vi "MAIN_HGB2.vi"() -> ()   [LabVIEW 2016]
uses:
  Producer_Case_Structure.ctl
  <vilib>/Utility/error.llb/DialogType.ctl
  <vilib>/express/express analysis/Spectral/Block/exnSpectralBlock spectral measurements RMS poly.vi
  <vilib>/express/express analysis/Spectral/Block/exnSpectralBlock spectral measurements RMS array WFM.vi
  <vilib>/express/express analysis/Spectral/XNode/ExpressSpectralMeasurementsBlockNode.xnode
panel:
  in  "Speed Setpoint":dbl
  in  "Operator Notes":string
  in  "Dummy Variable":dbl
  in  "Record Data":bool
  in  "Sample Rate [S/s]":dbl=10.0
  in  "file path":path=path "S:/002 - Projects/200804 AECSSB/6-Testing/TDMS Data/raw/080421-1"
  in  "Stop":bool=TRUE
  in  "Tab Control":T1(tab)=enum."Pressure & Temperature"
  out "System Temperatures":waveform(dbl)[](graph)=[{"t0"=timestamp(3710938237.209422 s since 1904-01-01), "dt"=0.1, "Y"=[25.06420596580779], "attributes"=variant("NI_ChannelName"=variant(string "T_dis"), "NI_UnitDescription"=variant(string "Deg C"))}, {"t0"=timestamp(3710938237.209422 s since 1904-01-01), "dt"=0.1, "Y"=[24.5131871952291], "attributes"=variant("NI_ChannelName"=variant(string "T_liq_mix"), "NI_UnitDescription"=variant(string "Deg C"))}, {"t0"=timestamp(3710938237.209422 s since 1904-01-01), "dt"=0.1, "Y"=[24.404692160048143], "attributes"=variant("NI_ChannelName"=variant(string "T_gas_mix"), "NI_UnitDescription"=variant(string "Deg C"))}, {"t0"=timestamp(3710938237.209422 s since 1904-01-01), "dt"=0.1, "Y"=[24.9517211018332], "attributes"=variant("NI_ChannelName"=variant(string "T_wf_cond_out"), "NI_UnitDescription"=variant(string "Deg C"))}, {"t0"=timestamp(3710938237.209422 s since 1904-01-01), "dt"=0.1, "Y"=[24.75846841874906], "attributes"=variant("NI_ChannelName"=variant(string "T_cf_in"), "NI_UnitDescription"=variant(string "Deg C"))}]
  out "Power Constituents":waveform(dbl)[](graph)=[{"t0"=timestamp(3710938237.209422 s since 1904-01-01), "dt"=0.1, "Y"=[-0.0627204059992863], "attributes"=variant("NI_ChannelName"=variant(string "Voltage"))}, {"t0"=timestamp(3710938237.209422 s since 1904-01-01), "dt"=0.1, "Y"=[-0.029340257114334634], "attributes"=variant("NI_ChannelName"=variant(string "Frequency"))}, {"t0"=timestamp(3710938237.0104485 s since 1904-01-01), "dt"=0.1, "Y"=[], "attributes"=variant("NI_ChannelName"=variant(string "Torque"))}]
  out "System Pressures":waveform(dbl)[](graph)=[{"t0"=timestamp(3710938237.209422 s since 1904-01-01), "dt"=0.1, "Y"=[653.0149804276925], "attributes"=variant("NI_ChannelName"=variant(string "P_comp_suc"))}, {"t0"=timestamp(3710938237.209422 s since 1904-01-01), "dt"=0.1, "Y"=[652.9848572024544], "attributes"=variant("NI_ChannelName"=variant(string "P_comp_dis"))}, {"t0"=timestamp(3710938237.209422 s since 1904-01-01), "dt"=0.1, "Y"=[653.0856354357659], "attributes"=variant("NI_ChannelName"=variant(string "P_comp_int"))}]
  out "Mass Flow":waveform(dbl)(graph)={"t0"=timestamp(3710938237.209422 s since 1904-01-01), "dt"=0.1, "Y"=[-2.0362630357040334e-05], "attributes"=variant("NI_ChannelName"=variant(string "m_dot_wf"))}
  out "Raw Acceleration":waveform(dbl)[](graph)
  out "Accel. Spectrum":cluster{"f0":dbl, "df":dbl, "magnitude":dbl[]}[](graph)
  in  "?":path=path "C:/Users/ASITest/Desktop/REFPROP"
  in  "Working Fluid":string="R134A.FLD"
  out "Sound":waveform(dbl)(graph)
  in  "Range":enum16{"40-70 dB", "auto", "60-90 dB"}(ring)
  in  "Ambient Noise [dB]":dbl=74.0
  # "Stop VI"
  # "Air Squared Hot Gas Bypass Test Stand"
  # "Point to where REFPROP is..."
  # "Registar Index of Calc Characteristics"
  # "INPUT NEEDED"
  # "0 = No\n1 = Yes"
  # "0 = No\n1 = Yes"
  # "UNITS:\nkg/s\nC\nRPM\nkPa\nV\nA"
  # "... where is the sensor in the initialization indexing?"
  # "Must have sound meter set up to manual range:\n1. click 'RNG' button on the meter \n2. the value displayed under 'SPL' on the display is the min of the range\n3. ensure the meter is on 'FAST' mode by clicking 'F/S', 'FAST' will be read on display\n4. use the A/C to select 'A' mode displayed on meter\n5. BEFORE INITIALIZING - set ambient noise level to whatever the sensor measures before running\n* the extech 407730 display frequency is not as high as the display freq here, so peak values\nmay not be seen on the sound meter display."
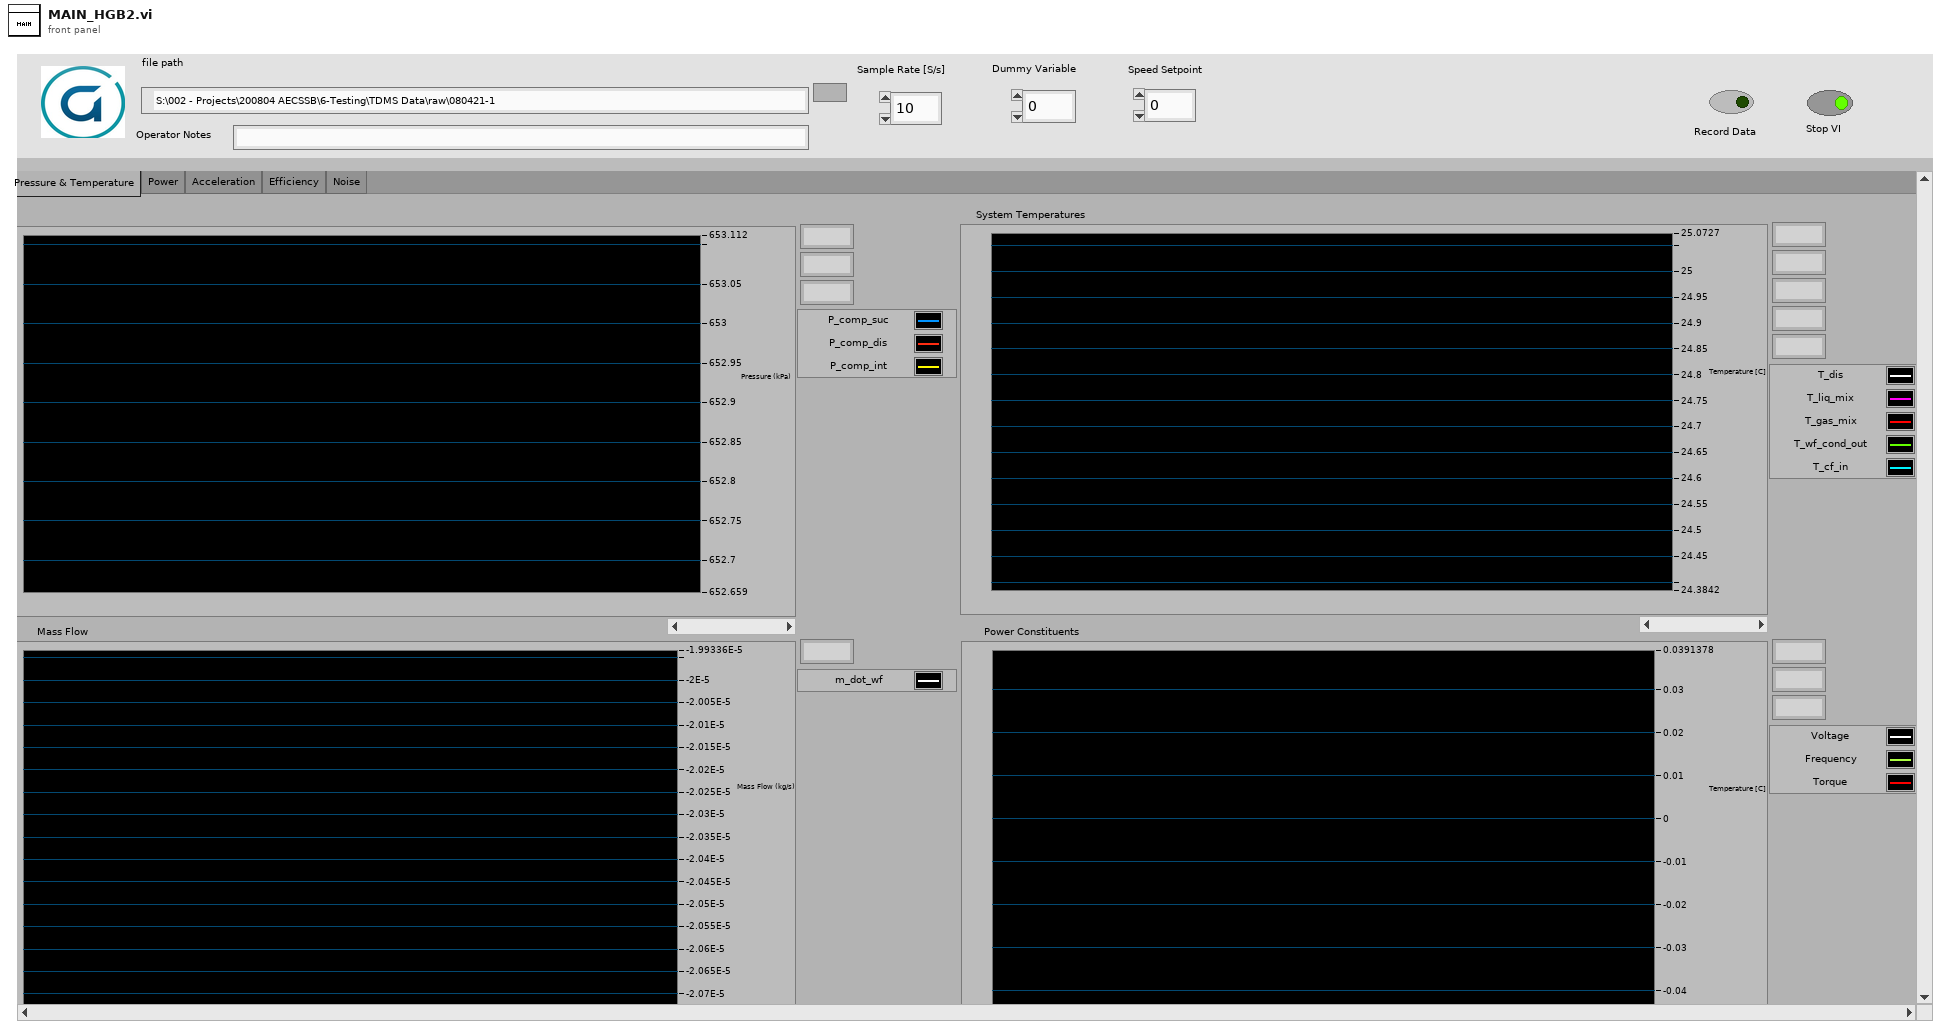
[diagram p1: front panel]
types:
  T1 = enum32{"Schematic", "Pressure & Temperature", "Power", "Acceleration", "Efficiency", "Noise"}
  T2 = enum16{"open", "open or create", "create or replace", "create", "open (read-only)"}
  T3 = typedef "Producer_Case_Structure.ctl" = enum16{"Initialize", "Read", "Write", "Display", "Queue", "Error"}
  T4 = cluster{"Data Main":waveform(dbl)[], "Accelerometer":waveform(dbl)[], "Dummy Variable":dbl, "Operator Notes":string, "RMS Current [A]":dbl, "Sound":waveform(dbl)[], "Eff. Data":waveform(dbl)[], "NI 6001":waveform(dbl)[], "Speed Setpoint":dbl}
  T5 = typedef "DialogType.ctl" = u16
  T6 = cluster{"averaging mode":u16, "weighting mode":u16, "number of averages":u32}
  T7 = cluster{"dB On (F)":bool, "unwrap phase (F)":bool, "convert to degree (F)":bool}
  T8 = cluster{"All Channels":tag[], "All Labels":string[], "All Units":string[], "Slope":dbl[], "Y-Intercept":dbl[]}
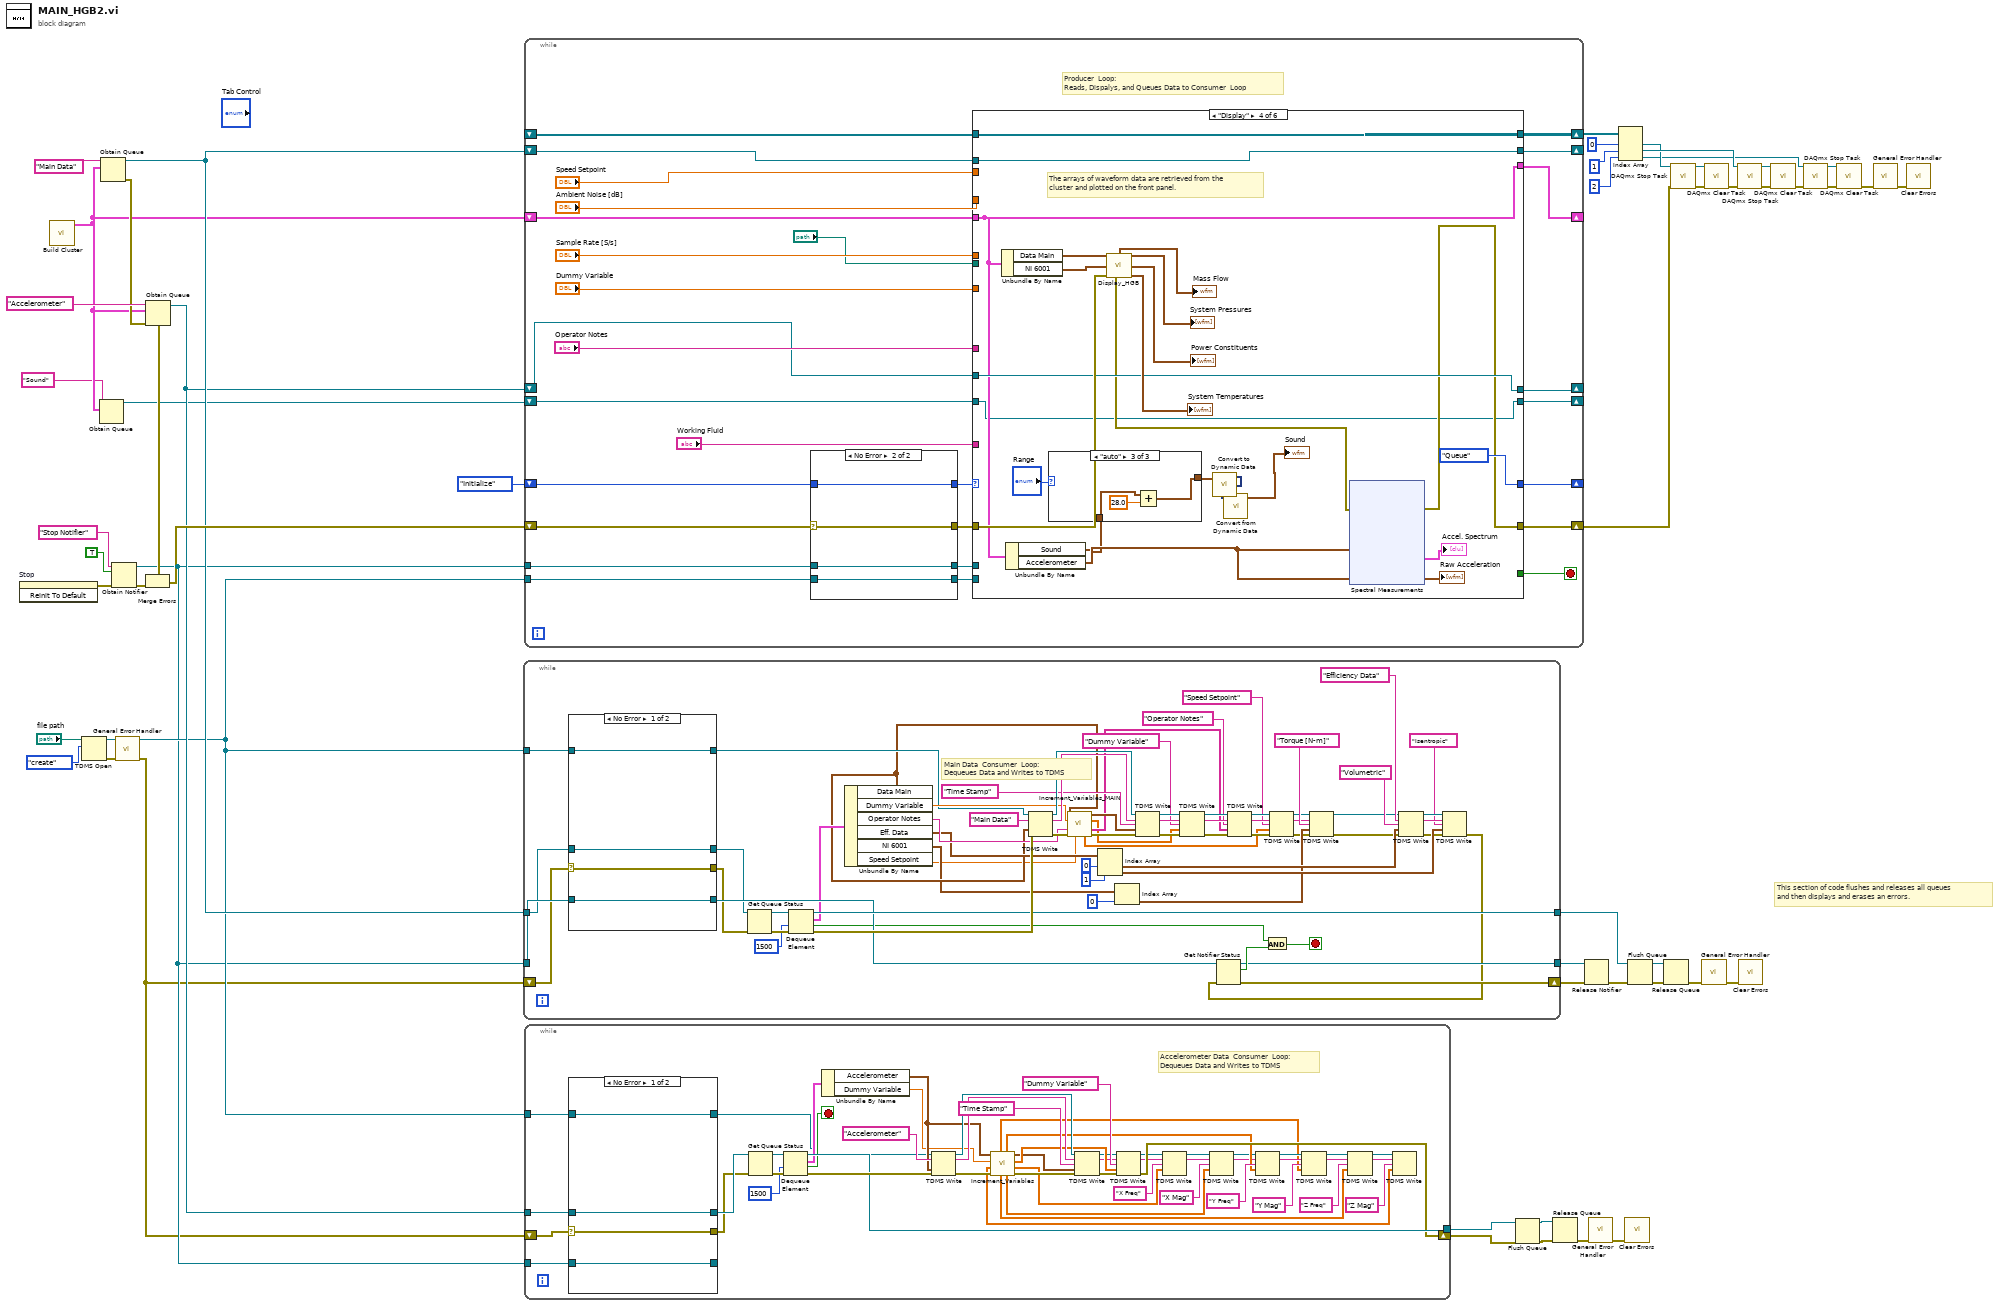
[diagram p0: block diagram]
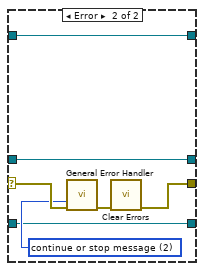
[diagram p2: hidden frame]
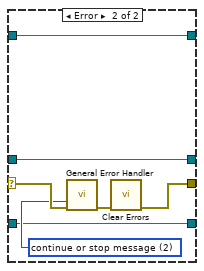
[diagram p3: hidden frame]
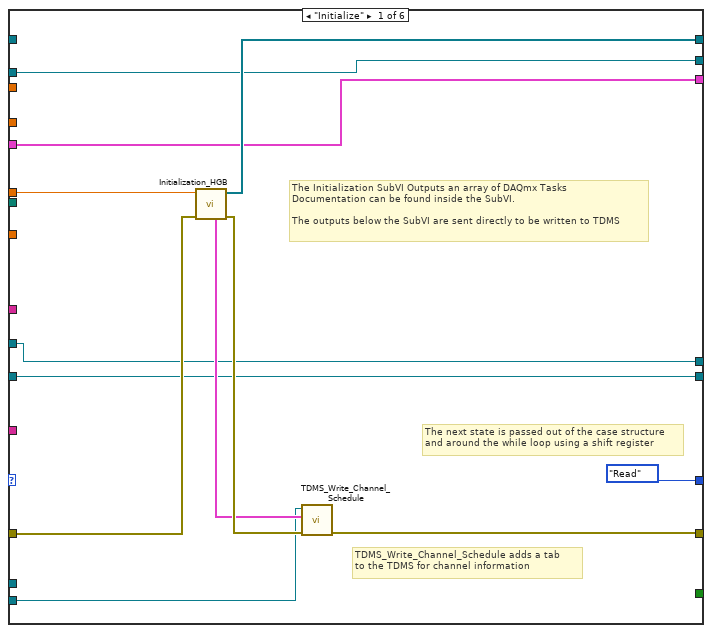
[diagram p4: hidden frame]
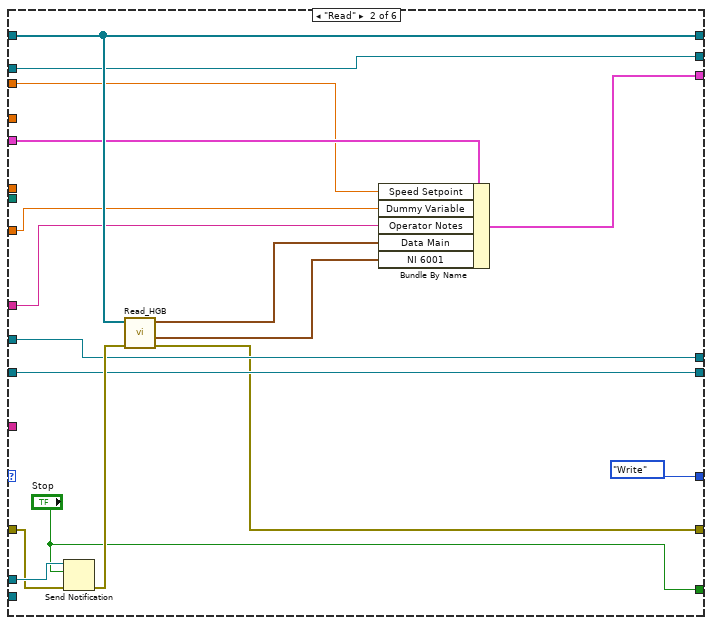
[diagram p5: hidden frame]
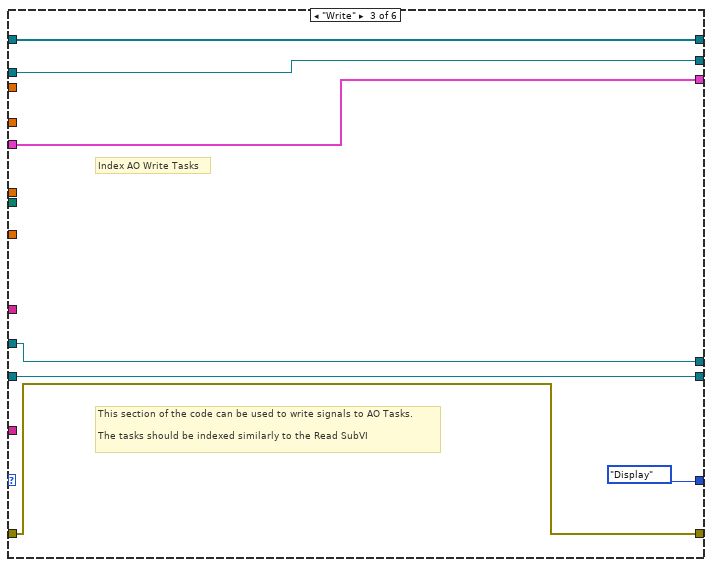
[diagram p6: hidden frame]
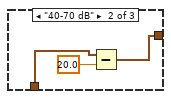
[diagram p8: hidden frame]
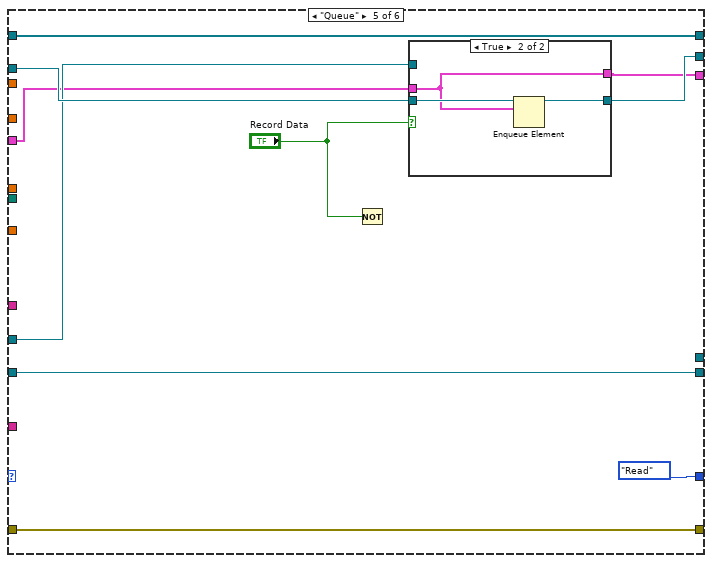
[diagram p9: hidden frame]
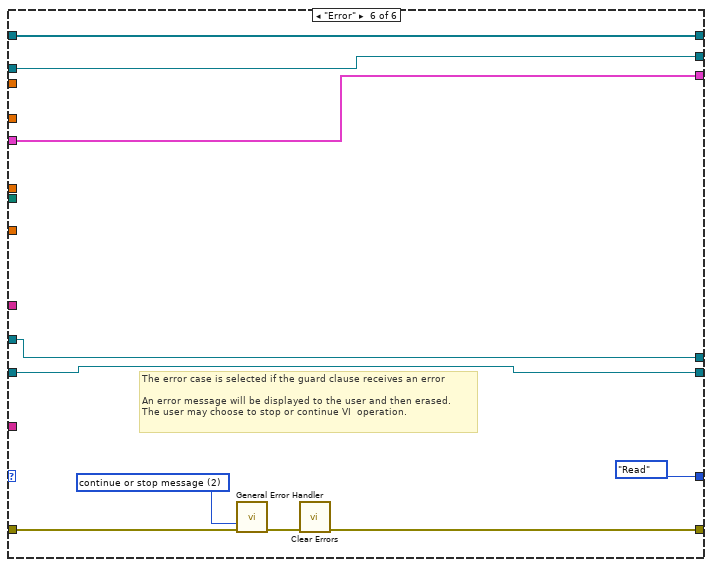
[diagram p11: hidden frame]
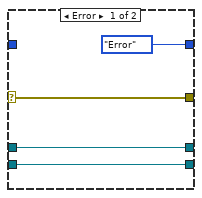
[diagram p12: hidden frame]
diagram:
  # "This section of code flushes and releases all queues \nand then displays and erases an errors."
  n1 = invoke on="Stop" class="Bool (strict)" method="Reinit To Default"() -> (error out=w47:errorcluster)  [unwired: 3 in, 2 out]
  n2 = call "Build Cluster.vi"() -> ("output cluster"=w15:T4)  [unwired: 11 in]
  n3 = TDMS Open(10:T2."create" ("operation (0:open)"), 11:"file path") -> (0:w40:errorcluster, 3:w11:refnum<k34>)  [unwired: 5 in]
  n4 = Obtain Queue(name (unnamed)="Sound", element data type=w15) -> (queue out=w12:refnum<queue>)  [unwired: 3 in, 2 out]
  n5 = Obtain Queue(name (unnamed)="Main Data", element data type=w15) -> (queue out=w37:refnum<queue>, error out=w23:errorcluster)  [unwired: 3 in, 1 out]
  n6 = Obtain Notifier(name (unnamed)="Stop Notifier", notification data type=TRUE, error in (no error)=w47) -> (notifier out=w10:refnum<notifier>, error out=w38:errorcluster)  [unwired: 1 in, 1 out]
  n7 = call <vilib>:"General Error Handler.vi"("error in (no error)"=w40) -> ("error out"=w8:errorcluster)  [unwired: 10 in, 4 out]
  n8 = Obtain Queue(name (unnamed)="Accelerometer", element data type=w15, error in (no error)=w23) -> (queue out=w21:refnum<queue>, error out=w22:errorcluster)  [unwired: 2 in, 1 out]
  n9 = Merge Errors(w22, w38) -> (w53:errorcluster)
  n10 = while {
    tunnel: w11 -> [w107]
    tunnel: [w117] -> w35
    tunnel: w37 -> [w108]
    tunnel: w10 -> [w110]
    shift-right: [w115] -> w32
    shift-left: w8 -> [w106]
    tunnel: [w85] -> w30
    stop <- w112 stop-if-true
    # "Main Data  Consumer  Loop: \nDequeues Data and Writes to TDMS"
    n11 = case shown="No Error" w106 {
      selector: w106 -> [w123 w129]
      tunnel: [w123 w128] -> w88
      tunnel: w110 -> [w122 w124]
      tunnel: [w122 w124] -> w111
      tunnel: [w121 w126] -> w109
      tunnel: w108 -> [w121 w126]
      tunnel: [w120 w125] -> w86
      tunnel: w107 -> [w120 w125]
      frame No Error {
      }
      frame Error {
        w127 = T5 2 items=["no dialog", "OK message", "continue or stop message", "OK message + warnings", "continue/stop + warnings"] ("type of dialog (OK msg:1)")
        n12 = call <vilib>:"General Error Handler.vi"("type of dialog (OK msg:1)"=w127, "error in (no error)"=w129) -> ("error out"=w130:errorcluster)  [unwired: 9 in, 4 out]
        n13 = call <vilib>:"Clear Errors.vi"("error in (no error)"=w130) -> ("error out"=w128:errorcluster)  [unwired: 5 in, 1 out]
      }
    }
    n14 = Get Queue Status(queue=w109, error in (no error)=w88) -> (queue out=w114:refnum<queue>, error out=w118:errorcluster)  [unwired: 1 in, 6 out]
    n15 = Dequeue Element(queue=w114, timeout in ms (-1)=1500, error in (no error)=w118) -> (queue out=w117:refnum<queue>, element=w87:T4, timed out?=w105:bool, error out=w119:errorcluster)
    n16 = Unbundle By Name(w87) -> ("Data Main"=w66:waveform(dbl)[], "Dummy Variable"=w95:dbl, "Operator Notes"=w83:string, "Eff. Data"=w67:waveform(dbl)[], "NI 6001"=w64:waveform(dbl)[], "Speed Setpoint"=w55:dbl)
    n17 = TDMS Write(0:w86, 5:"Main Data" ("group name in (Untitled)"), 9:w66, 11:w119) -> (4:w102:refnum<k34>, 6:w100:string, 15:w103:errorcluster)  [unwired: 2 in, 1 out]
    n18 = call "Increment_Variables_MAIN.vi"("Data Main"=w66, "Dummy Variable"=w95, "Operator Notes"=w83, "error in 2"=w103, "Speed Setpoint"=w55) -> ("Time Stamp"=w96:timestamp[], "Dummy Variable Array"=w54:dbl[], "Operator Notes Array"=w84:string[], "Speed Setpoint Array"=w79:dbl[], "error IO"=w104:errorcluster)  [unwired: 6 in]
    n19 = Index Array(array=w67, index #1=0 ("index"), index #2=1 ("index")) -> (element #1=w75:waveform(dbl), element #2=w72:waveform(dbl))
    n20 = Index Array(array=w64, index=0) -> (element=w60:waveform(dbl))
    n21 = TDMS Write(0:w102, 5:w100, 7:"Time Stamp" ("group name in (Untitled)"), 9:w96, 11:w104) -> (4:w99:refnum<k34>, 6:w97:string, 15:w98:errorcluster)  [unwired: 1 in, 1 out]
    n22 = TDMS Write(0:w99, 5:w97, 7:"Dummy Variable" ("group name in (Untitled)"), 9:w54, 11:w98) -> (4:w93:refnum<k34>, 6:w92:string, 15:w94:errorcluster)  [unwired: 1 in, 1 out]
    n23 = TDMS Write(0:w93, 5:w92, 7:"Operator Notes" ("group name in (Untitled)"), 9:w84, 11:w94) -> (4:w80:refnum<k34>, 6:w81:string, 15:w82:errorcluster)  [unwired: 1 in, 1 out]
    n24 = TDMS Write(0:w80, 5:w81, 7:"Speed Setpoint" ("group name in (Untitled)"), 9:w79, 11:w82) -> (4:w62:refnum<k34>, 6:w61:string, 15:w59:errorcluster)  [unwired: 1 in, 1 out]
    n25 = TDMS Write(0:w62, 5:w61, 7:"Torque [N-m]" ("channel name(s) in (Untitled)"), 9:w60, 11:w59) -> (4:w58:refnum<k34>, 15:w57:errorcluster)  [unwired: 1 in, 2 out]
    n26 = TDMS Write(0:w58, 5:"Efficiency Data" ("group name in (Untitled)"), 7:"Volumetric" ("channel name(s) in (Untitled)"), 9:w75, 11:w57) -> (4:w71:refnum<k34>, 6:w70:string, 15:w68:errorcluster)  [unwired: 1 in, 1 out]
    n27 = TDMS Write(0:w71, 5:w70, 7:"Isentropic" ("channel name(s) in (Untitled)"), 9:w72, 11:w68) -> (15:w56:errorcluster)  [unwired: 1 in, 3 out]
    n28 = Get Notifier Status(notifier=w111, error in (no error)=w56) -> (notifier out=w85:refnum<notifier>, current notification=w116:bool, error out=w115:errorcluster)  [unwired: 2 out]
    n29 = And(x=w105, y=w116) -> (x .and. y?=w112:bool)
  }
  n30 = while {
    shift-right: [w151] -> _
    shift-left: Producer_Case_Structure."Initialize" ("Enum") -> [w157]
    shift-right: [w153] -> w43
    shift-left: _ -> [w152]
    tunnel: w10 -> [w158]
    shift-right: [w148] -> _
    shift-left: w15 -> [w147]
    shift-right: [w145] -> _
    shift-left: w37 -> [w144]
    shift-right: [w154] -> w44
    shift-left: w53 -> [w146]
    tunnel: w11 -> [w139]
    shift-right: [w137] -> _
    shift-left: w21 -> [w138]
    shift-right: [w136] -> _
    shift-left: w12 -> [w135]
    stop <- w150 stop-if-true
    # "Producer  Loop: \nReads, Dispalys, and Queues Data to Consumer  Loop"
    n31 = case shown="No Error" w146 {
      selector: w146 -> [w260 w266]
      tunnel: [w260 w266] -> w155
      tunnel: w158 -> [w262 w265]
      tunnel: [w262 w265] -> w149
      tunnel: w157 -> [_ w264]
      tunnel: [Producer_Case_Structure."Error" ("Enum") w264] -> w156
      tunnel: [w259 w263] -> w140
      tunnel: w139 -> [w259 w263]
      frame Error {
      }
      frame No Error {
      }
    }
    n32 = case shown="\"Display\"" w156 {
      tunnel: w155 -> [w170 w182 w189 w216 w241 w255]
      tunnel: [w163 w172 w189 w208 w241 w252] -> w154
      tunnel: [w169 w183 w194 w214 w242 w256] -> w153
      tunnel: w152 -> [_ w183 w194 w214 w242 w256]
      tunnel: [Producer_Case_Structure."Read" ("Enum") Producer_Case_Structure."Write" ("Enum") Producer_Case_Structure."Display" ("Enum") Producer_Case_Structure."Queue" ("Enum") Producer_Case_Structure."Read" ("Enum") Producer_Case_Structure."Read" ("Enum")] -> w151
      tunnel: [_ "Stop" _ _ _ _] -> w150
      tunnel: w149 -> [_ w185 _ _ _ _]
      tunnel: [w165 w180 w192 w207 w238 w254] -> w148
      tunnel: w147 -> [w165 w175 w192 w207 w236 w254]
      tunnel: [w167 w181 w191 w212 w239 w251] -> w145
      tunnel: w144 -> [w167 w181 w191 w212 w240 w251]
      tunnel: "Sample Rate [S/s]" -> [w166 _ _ _ _ _]
      tunnel: "Dummy Variable" -> [_ w177 _ _ _ _]
      tunnel: "Operator Notes" -> [_ w179 _ _ _ _]
      tunnel: w140 -> [w161 _ _ _ _ _]
      tunnel: w138 -> [w160 w178 w190 w210 w237 w250]
      tunnel: [w160 w178 w190 w210 _ w250] -> w137
      tunnel: [w159 w176 w188 w205 w235 w249] -> w136
      tunnel: w135 -> [w159 w176 w188 w205 w235 w249]
      tunnel: "Ambient Noise [dB]" -> [_ _ _ _ _ _]
      tunnel: "?" -> [_ _ _ _ _ _]
      tunnel: "Working Fluid" -> [_ _ _ _ _ _]
      tunnel: "Speed Setpoint" -> [_ w173 _ _ _ _]
      frame "Initialize" {
        # "TDMS_Write_Channel_Schedule adds a tab \nto the TDMS for channel information"
        # "The next state is passed out of the case structure \nand around the while loop using a shift register"
        # "The Initialization SubVI Outputs an array of DAQmx Tasks\nDocumentation can be found inside the SubVI.\n\nThe outputs below the SubVI are sent directly to be written to TDMS"
        n33 = call "Initialization_HGB.vi"("error in"=w170, "Sample Rate"=w166) -> ("error out"=w164:errorcluster, "Task Array"=w169:refnum<k21>[], "output cluster"=w162:T8)  [unwired: 7 in]
        n34 = call "TDMS_Write_Channel_Schedule.vi"("error in (no error)"=w164, "output cluster"=w162, "Refnum in"=w161) -> ("error out"=w163:errorcluster)  [unwired: 8 in]
      }
      frame "Read" {
        n35 = Send Notification(notification="Stop", notifier=w185, error in (no error)=w182) -> (error out=w187:errorcluster)  [unwired: 1 out]
        n36 = call "Read_HGB.vi"("error in (no error)"=w187, "Task Array"=w183) -> ("error out"=w172:errorcluster, "NI 6001"=w171:waveform(dbl)[], "Data Main"=w174:waveform(dbl)[])  [unwired: 7 in]
        n37 = Bundle By Name(cluster=w175, "Speed Setpoint"=w173, "Dummy Variable"=w177, "Operator Notes"=w179, "Data Main"=w174, "NI 6001"=w171) -> (w180:T4)
      }
      frame "Write" {
        # "This section of the code can be used to write signals to AO Tasks.\n\nThe tasks should be indexed similarly to the Read SubVI"
        # "Index AO Write Tasks"
      }
      frame "Display" {
        # "The arrays of waveform data are retrieved from the \ncluster and plotted on the front panel."
        n38 = Unbundle By Name(w207) -> ("Data Main"=w199:waveform(dbl)[], "NI 6001"=w195:waveform(dbl)[])
        n39 = Unbundle By Name(w207) -> ("Sound"=w204:waveform(dbl)[], "Accelerometer"=w206:waveform(dbl)[])
        "Raw Acceleration" <- w206
        n40 = case shown="\"auto\"" "Range" {
          tunnel: [w217 w218 w221] -> w202
          tunnel: w204 -> [w217 w219 w222]
          frame "60-90 dB" {
          }
          frame "40-70 dB" {
            n41 = Subtract(x=w219, y=20.0) -> (x-y=w218:waveform(dbl)[])
          }
          frame "auto" {
            n42 = Add(x=w222, y=28.0) -> (x+y=w221:waveform(dbl)[])
          }
        }
        n43 = call "Display_HGB.vi"("data"=w199, "NI 6001"=w195, "error in (no error)"=w216) -> ("Mass Flow"=→"Mass Flow":waveform(dbl), "System Pressures"=→"System Pressures":waveform(dbl)[], "Power Constituents"=→"Power Constituents":waveform(dbl)[], "error out"=w209:errorcluster, "System Temperatures"=→"System Temperatures":waveform(dbl)[])  [unwired: 8 in]
        n44 = call "Convert to Dynamic Data"("Array of Waveforms"=w202) -> ("Dynamic Data Type"=w200:dynamicdata)  [unwired: 3 in]
        n45 = call "Convert from Dynamic Data"("Dynamic Data Type"=w200) -> ("Waveform"=→"Sound":waveform(dbl))  [unwired: 3 in]
        n46 = xnode "Spectral Measurements"("Signals"=w206, "error in (no error)"=w209) -> ("FFT - (RMS)"=→"Accel. Spectrum":cluster{"f0":dbl, "df":dbl, "magnitude":dbl[]}[], "error out"=w208:errorcluster)  [unwired: 1 out]
      }
      frame "Queue" {
        n47 = Not(x="Record Data") -> ()  [unwired: 1 out]
        n48 = case shown="True" "Record Data" {
          tunnel: w236 -> [w244 w246]
          tunnel: w240 -> [w245 w247]
          tunnel: [w245 w248] -> w239
          tunnel: [w244 w246] -> w238
          tunnel: w237 -> [_ _]
          frame False {
          }
          frame True {
            n49 = Enqueue Element(queue=w247, element=w246) -> (queue out=w248:refnum<queue>)  [unwired: 2 in, 2 out]
          }
        }
      }
      frame "Error" {
        w257 = T5 2 items=["no dialog", "OK message", "continue or stop message", "OK message + warnings", "continue/stop + warnings"] ("type of dialog (OK msg:1)")
        # "The error case is selected if the guard clause receives an error\n\nAn error message will be displayed to the user and then erased. \nThe user may choose to stop or continue VI  operation."
        n50 = call <vilib>:"General Error Handler.vi"("type of dialog (OK msg:1)"=w257, "error in (no error)"=w255) -> ("error out"=w253:errorcluster)  [unwired: 9 in, 4 out]
        n51 = call <vilib>:"Clear Errors.vi"("error in (no error)"=w253) -> ("error out"=w252:errorcluster)  [unwired: 5 in, 1 out]
      }
    }
  }
  n52 = while {
    tunnel: w11 -> [w311]
    tunnel: [w317] -> w16
    tunnel: w21 -> [w312]
    tunnel: w10 -> [w314]
    shift-right: [w292] -> w9
    shift-left: w8 -> [w310]
    stop <- w291 stop-if-true
    # "Accelerometer Data  Consumer  Loop: \nDequeues Data and Writes to TDMS"
    n53 = case shown="No Error" w310 {
      selector: w310 -> [w323 w329]
      tunnel: [w323 w328] -> w302
      tunnel: w314 -> [w322 w324]
      tunnel: [w322 w324] -> _
      tunnel: [w321 w326] -> w313
      tunnel: w312 -> [w321 w326]
      tunnel: [w320 w325] -> w300
      tunnel: w311 -> [w320 w325]
      frame No Error {
      }
      frame Error {
        w327 = T5 2 items=["no dialog", "OK message", "continue or stop message", "OK message + warnings", "continue/stop + warnings"] ("type of dialog (OK msg:1)")
        n54 = call <vilib>:"General Error Handler.vi"("type of dialog (OK msg:1)"=w327, "error in (no error)"=w329) -> ("error out"=w330:errorcluster)  [unwired: 9 in, 4 out]
        n55 = call <vilib>:"Clear Errors.vi"("error in (no error)"=w330) -> ("error out"=w328:errorcluster)  [unwired: 5 in, 1 out]
      }
    }
    n56 = Get Queue Status(queue=w313, error in (no error)=w302) -> (queue out=w316:refnum<queue>, error out=w318:errorcluster)  [unwired: 1 in, 6 out]
    n57 = Dequeue Element(queue=w316, timeout in ms (-1)=1500, error in (no error)=w318) -> (queue out=w317:refnum<queue>, element=w301:T4, timed out?=w291:bool, error out=w319:errorcluster)
    n58 = Unbundle By Name(w301) -> ("Accelerometer"=w304:waveform(dbl)[], "Dummy Variable"=w299:dbl)
    n59 = TDMS Write(0:w300, 5:"Accelerometer" ("group name in (Untitled)"), 9:w304, 11:w319) -> (4:w307:refnum<k34>, 6:w305:string, 15:w308:errorcluster)  [unwired: 2 in, 1 out]
    n60 = call "Increment_Variables.vi"("error in 2"=w308, "Dummy Variable"=w299, "Accelerometer"=w304) -> ("error IO"=w309:errorcluster, "X Accel Freq Array"=w288:dbl[], "Dummy Variable Array"=w297:dbl[], "Time Stamp"=w293:timestamp[], "X Accel Mag Array"=w286:dbl[], "Y Accel Freq Array"=w269:dbl[], "Z Accel Freq Array"=w271:dbl[], "Y Accel Mag Array"=w270:dbl[], "Z Accel Mag Array"=w272:dbl[])
    n61 = TDMS Write(0:w307, 5:w305, 7:"Time Stamp" ("group name in (Untitled)"), 9:w293, 11:w309) -> (4:w294:refnum<k34>, 6:w295:string, 15:w298:errorcluster)  [unwired: 1 in, 1 out]
    n62 = TDMS Write(0:w294, 5:w295, 7:"Dummy Variable" ("group name in (Untitled)"), 9:w297, 11:w298) -> (4:w289:refnum<k34>, 6:w290:string, 15:w292:errorcluster)  [unwired: 1 in, 1 out]
    n63 = TDMS Write(0:w289, 5:w290, 7:"X Freq" ("group name in (Untitled)"), 9:w288) -> (4:w283:refnum<k34>, 6:w284:string)  [unwired: 2 in, 2 out]
    n64 = TDMS Write(0:w283, 5:w284, 7:"X Mag" ("group name in (Untitled)"), 9:w286) -> (4:w268:refnum<k34>, 6:w267:string)  [unwired: 2 in, 2 out]
    n65 = TDMS Write(0:w268, 5:w267, 7:"Y Freq" ("group name in (Untitled)"), 9:w269) -> (4:w280:refnum<k34>, 6:w279:string)  [unwired: 2 in, 2 out]
    n66 = TDMS Write(0:w280, 5:w279, 7:"Y Mag" ("group name in (Untitled)"), 9:w270) -> (4:w281:refnum<k34>, 6:w282:string)  [unwired: 2 in, 2 out]
    n67 = TDMS Write(0:w281, 5:w282, 7:"Z Freq" ("group name in (Untitled)"), 9:w271) -> (4:w278:refnum<k34>, 6:w277:string)  [unwired: 2 in, 2 out]
    n68 = TDMS Write(0:w278, 5:w277, 7:"Z Mag" ("group name in (Untitled)"), 9:w272) -> ()  [unwired: 2 in, 4 out]
  }
  n69 = Flush Queue(queue=w16, error in (no error)=w9) -> (queue out=w19:refnum<queue>, error out=w18:errorcluster)  [unwired: 1 out]
  n70 = Release Queue(queue=w19, error in (no error)=w18) -> (error out=w17:errorcluster)  [unwired: 1 in, 2 out]
  n71 = Release Notifier(notifier=w30, error in (no error)=w32) -> (error out=w31:errorcluster)  [unwired: 1 in, 2 out]
  n72 = call <vilib>:"General Error Handler.vi"("error in (no error)"=w17) -> ("error out"=w20:errorcluster)  [unwired: 10 in, 4 out]
  n73 = Index Array(array=w43, index #1=0 ("index"), index #2=1 ("index"), index #3=2 ("index")) -> (element #1=w6:refnum<k21>, element #2=w27:refnum<k21>, element #3=w1:refnum<k21>)
  n74 = call <vilib>:"Clear Errors.vi"("error in (no error)"=w20) -> ()  [unwired: 5 in, 2 out]
  n75 = Flush Queue(queue=w35, error in (no error)=w31) -> (queue out=w36:refnum<queue>, error out=w34:errorcluster)  [unwired: 1 out]
  n76 = Release Queue(queue=w36, error in (no error)=w34) -> (error out=w33:errorcluster)  [unwired: 1 in, 2 out]
  n77 = call <vilib>:"DAQmx Stop Task.vi"("task/channels in"=w6, "error in"=w44) -> ("task out"=w45:refnum<k21>, "error out"=w46:errorcluster)  [unwired: 12 in]
  n78 = call <vilib>:"General Error Handler.vi"("error in (no error)"=w33) -> ("error out"=w41:errorcluster)  [unwired: 10 in, 4 out]
  n79 = call <vilib>:"DAQmx Clear Task.vi"("task in"=w45, "error in"=w46) -> ("error out"=w28:errorcluster)  [unwired: 13 in]
  n80 = call <vilib>:"DAQmx Stop Task.vi"("task/channels in"=w27, "error in"=w28) -> ("task out"=w25:refnum<k21>, "error out"=w29:errorcluster)  [unwired: 12 in]
  n81 = call <vilib>:"Clear Errors.vi"("error in (no error)"=w41) -> ()  [unwired: 5 in, 2 out]
  n82 = call <vilib>:"DAQmx Clear Task.vi"("task in"=w25, "error in"=w29) -> ("error out"=w3:errorcluster)  [unwired: 13 in]
  n83 = call <vilib>:"DAQmx Stop Task.vi"("task/channels in"=w1, "error in"=w3) -> ("task out"=w4:refnum<k21>, "error out"=w5:errorcluster)  [unwired: 12 in]
  n84 = call <vilib>:"DAQmx Clear Task.vi"("task in"=w4, "error in"=w5) -> ("error out"=w2:errorcluster)  [unwired: 13 in]
  n85 = call <vilib>:"General Error Handler.vi"("error in (no error)"=w2) -> ("error out"=w13:errorcluster)  [unwired: 10 in, 4 out]
  n86 = call <vilib>:"Clear Errors.vi"("error in (no error)"=w13) -> ()  [unwired: 5 in, 2 out]
